vi "convert channel number into DAQ channel string.vi"(10 "Numeric":u8) -> (2 "String":string)   [LabVIEW 2015]
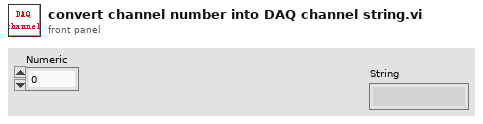
[diagram p1: front panel]
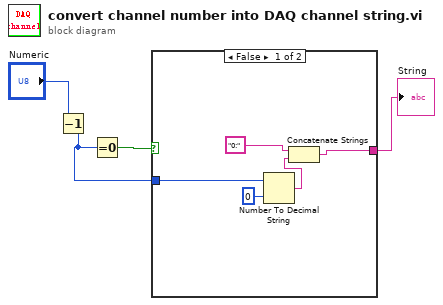
[diagram p0: block diagram]
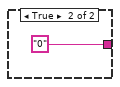
[diagram p2: hidden frame]
diagram:
  n1 = Decrement(x="Numeric") -> (x-1=w1:u8)
  n2 = Equal To 0?(x=w1) -> (x = 0?=w4:bool)
  n3 = case shown="False" w4 {
    tunnel: [w5 "0"] -> w3
    tunnel: w1 -> [w6 _]
    frame False {
      n4 = Number To Decimal String(number=w6, width (-)=i16 0) -> (decimal integer string=w8:string)
      n5 = Concatenate Strings("0:", w8) -> (w5:string)
    }
    frame True {
    }
  }
  "String" <- w3
